vi "Merge_into_Array_double.vi"(1 "Index":i32, 2 "Insert":dbl, 3 "1D Array":dbl[](array[numeric]), 4 "2D Array":dbl[][](array[numeric])) -> (0 "Output Array":dbl[][](array[numeric]))   [LabVIEW 2015]
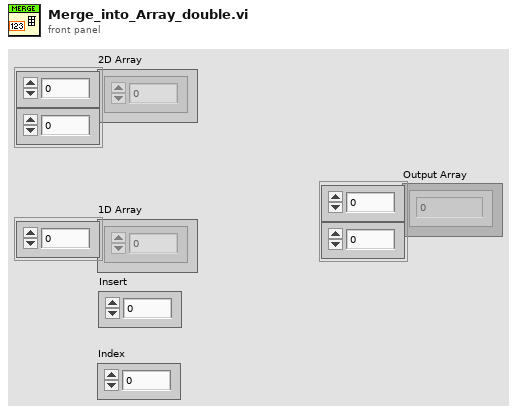
[diagram p1: front panel]
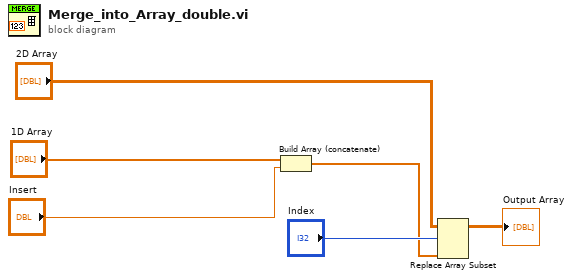
[diagram p0: block diagram]
diagram:
  n1 = Build Array (concatenate)("1D Array", "Insert") -> (w2:dbl[])
  n2 = Replace Array Subset(array="2D Array", new element=w2, index (row)="Index") -> (→"Output Array":dbl[][])  [unwired: 1 in]
